vi "I²C-lsm303agr.vi"() -> ()   [LabVIEW 2019]
panel:
  out "Numeric 3":i16
  in  "Numeric 2":i16
  in  "Numeric":i16
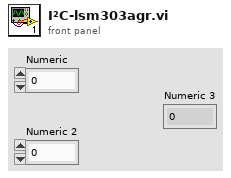
[diagram p1: front panel]
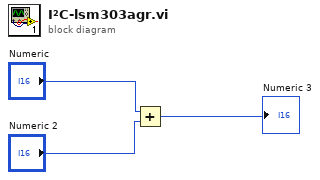
[diagram p0: block diagram]
diagram:
  n1 = Add(x="Numeric", y="Numeric 2") -> (x+y=→"Numeric 3":i16)
